vi "LIA.TestLauncher.vi"() -> ()   [LabVIEW 2017, in "LIA.lvclass"]
doc: "JKI State Machine Objects (SMO) 1.0.0.5\nJKI - JKI\nCopyright (c) 2016, JKI"
uses:
  LIA.lvclass
  <vilib>/JKI/JKI SMO/SMO/Typedefs/SMOState --Enum.ctl
  D:/Program Files (x86)/National Instruments/LabVIEW 2017/vi.lib/JKI/JKI SMO/SMO/SMO.lvclass
  <vilib>/JKI/JKI SMO/SMO/SMO.lvclass
panel:
  out "Array":T1[](array[typedef])
  out "SMO State":T1
  out "error out":errorcluster
  in  "Stop":bool
  # "SMO Test Launcher"
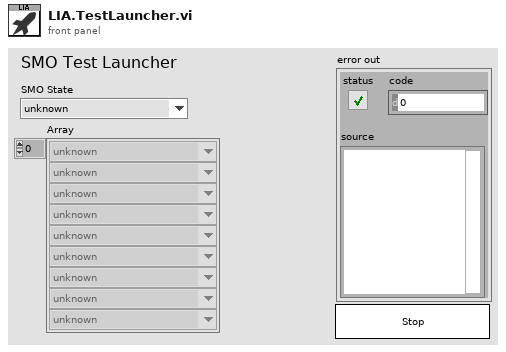
[diagram p1: front panel]
types:
  T1 = typedef "SMO.lvclass/SMOState --Enum.ctl" = enum16{"unknown", "Created", "Started", "Stopped"}
  T2 = typedef "SMO.lvclass/Public Events.ctl" = cluster{"Error":refnum<user-event>, "State":refnum<user-event>, "Reserve State":refnum<user-event>}
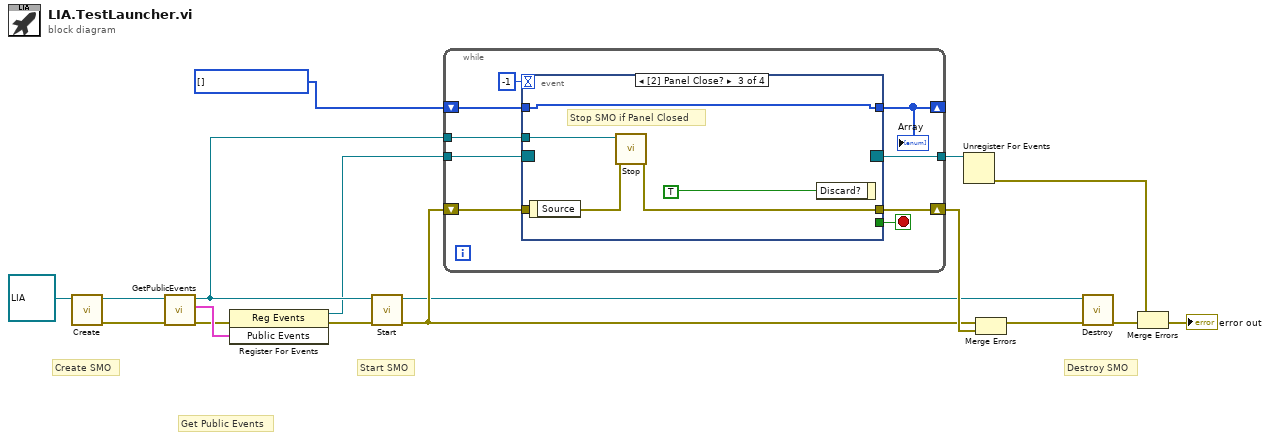
[diagram p0: block diagram]
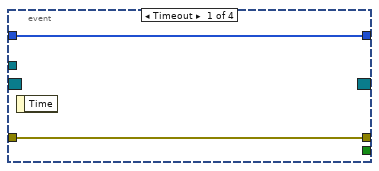
[diagram p2: hidden frame]
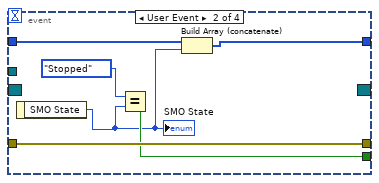
[diagram p3: hidden frame]
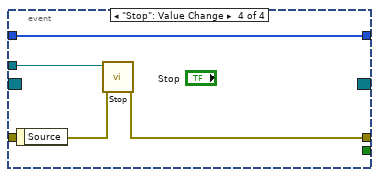
[diagram p4: hidden frame]
diagram:
  w1 = T1[] [] items=["unknown", "Created", "Started", "Stopped"]
  # "Get Public Events"
  # "Start SMO"
  # "Destroy SMO"
  # "Create SMO"
  n1 = call <vilib>:"Create.vi"("SMO"=refnum<class "LIA.lvclass"> refnum ("SMO.Template.lvclass")) -> ("error out"=w2:errorcluster, "SMO out"=w3:refnum<class "LIA.lvclass">)  [unwired: 8 in, 1 out]
  n2 = call <vilib>:"GetPublicEvents.vi"("error in (no error)"=w2, "SMO"=w3) -> ("error out"=w5:errorcluster, "Public Events"=w6:T2, "SMO out"=w8:refnum<class "LIA.lvclass">)  [unwired: 7 in]
  n3 = register-events(error in=w5, w6) -> (reference out=w4:refnum<event-registration>, error out=w7:errorcluster)  [unwired: 1 in]
  n4 = call <vilib>:"Start.vi"("error in (no error)"=w7, "SMO"=w8) -> ("error out"=w11:errorcluster, "SMO out"=w9:refnum<class "LIA.lvclass">)  [unwired: 8 in]
  n5 = while {
    shift-right: [w25] -> w16
    shift-left: w11 -> [w24]
    tunnel: w4 -> [w23]
    tunnel: [w22] -> w17
    tunnel: w8 -> [w21]
    shift-right: [w18] -> _
    shift-left: w1 -> [w19]
    stop <- w26 stop-if-true
    n6 = event shown="[2] Panel Close?" {
      selector: w23 -> [_ _ _ _]
      dyn-events: [_ _ _ _] -> w22
      timeout: -1 -> [_ _ _ _]
      tunnel: [_ w32 _ _] -> w26
      tunnel: w21 -> [_ _ w39 w43]
      tunnel: [w28 w34 w38 w42] -> w25
      tunnel: w24 -> [w28 w34 w37 w41]
      tunnel: w19 -> [w27 w31 w35 w40]
      tunnel: [w27 w29 w35 w40] -> w18
      event Timeout {
        n7 = event-data() -> ()  [unwired: 1 in, 1 out]
      }
      event User Event {
        n8 = event-data() -> ("SMO State"=w30:T1)  [unwired: 1 in]
        "SMO State" <- w30
        n9 = Equal?(x=SMOState_--Enum."Stopped", y=w30) -> (x = y?=w32:bool)
        n10 = Build Array (concatenate)(w31, w30) -> (w29:T1[])
      }
      event Panel Close? {
        # "Stop SMO if Panel Closed"
        n11 = event-data() -> ()  [unwired: 1 in, 1 out]
        n12 = call <vilib>:"Stop.vi"("error in (no error)"=w37, "SMO"=w39) -> ("error out"=w38:errorcluster)  [unwired: 8 in, 1 out]
        n13 = event-data("Discard?"=TRUE ("OK")) -> ()  [unwired: 1 in, 1 out]
      }
      event "Stop": Value Change {
        n14 = event-data() -> ()  [unwired: 1 in, 1 out]
        n15 = call <vilib>:"Stop.vi"("error in (no error)"=w41, "SMO"=w43) -> ("error out"=w42:errorcluster)  [unwired: 8 in, 1 out]
      }
    }
    "Array" <- w18
  }
  n16 = Unregister For Events(event registration refnum=w17) -> (error out=w15:errorcluster)  [unwired: 1 in]
  n17 = Merge Errors(w11, w16) -> (w10:errorcluster)
  n18 = call <vilib>:"Destroy.vi"("error in (no error)"=w10, "SMO"=w9) -> ("error out"=w13:errorcluster)  [unwired: 9 in]
  n19 = Merge Errors(w15, w13) -> (→"error out":errorcluster)
